vi "DisplayErrorsForDevice.vi"(0 "CmdLib In":refnum<k24>, 1 "Device Key":string, 2 "Device Address":i32, 3 "Prefix":string, 4 "Status:":refnum<vi>, 5 "error in":errorcluster) -> (14 "CmdLib Out":refnum<k24>, 15 "DeviceKey Out":string, 16 "Device Address Out":i32, 19 "error out":errorcluster)   [LabVIEW 2019]
uses:
  C:/Users/jyxks/OneDrive/Documents/Program Files/New Focus/New Focus Picomotor Application/Samples/LabVIEW/Model 8742/LabVIEW 2009/CmdLib.dll
  Program Files/New Focus/New Focus Picomotor Application/Samples/LabVIEW/Model 8742/LabVIEW 2009/CmdLib.dll
  <vilib>/regexp/Match Regular Expression.xnode
panel:
  in  "errMsg":string
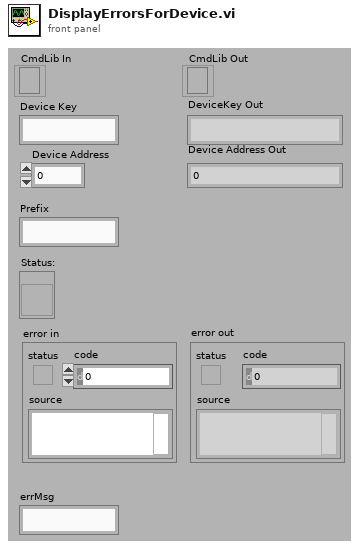
[diagram p1: front panel]
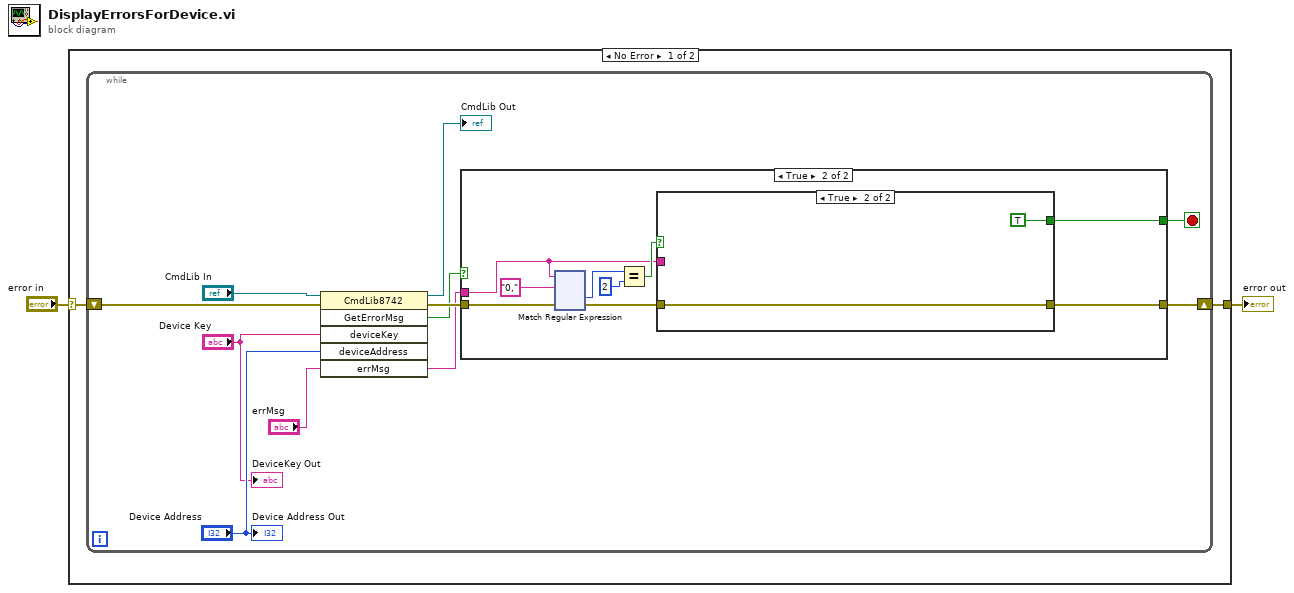
[diagram p0: block diagram]
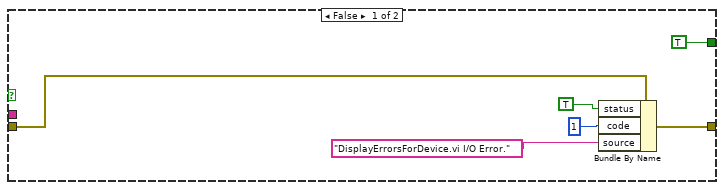
[diagram p2: hidden frame]
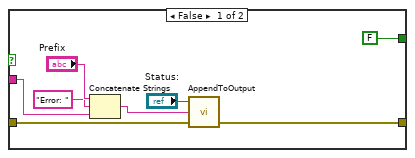
[diagram p3: hidden frame]
diagram:
  n1 = case shown="No Error" "error in" {
    selector: "error in" -> [w4 w155]
    tunnel: [w3 w155] -> w1
    frame No Error {
      n2 = while {
        shift-right: [w12] -> w3
        shift-left: w4 -> [w13]
        stop <- w5 stop-if-true
        n3 = invoke class="CmdLib8742" method="GetErrorMsg"(reference="CmdLib In", error in=w13, "deviceKey"="Device Key", "deviceAddress"="Device Address", "errMsg"="errMsg") -> (reference out=→"CmdLib Out":refnum<k24>, error out=w14:errorcluster, "GetErrorMsg"=w6:bool, "errMsg"=w7:string)  [unwired: 1 in, 2 out]
        n4 = case shown="True" w6 {
          tunnel: w14 -> [w21 w27]
          tunnel: [w16 w22] -> w12
          tunnel: w7 -> [_ w23]
          tunnel: [TRUE w25] -> w5
          frame False {
            n5 = Bundle By Name(cluster=w21, "status"=TRUE, "code"=1, "source"="DisplayErrorsForDevice.vi I/O Error.") -> (w16:errorcluster)
          }
          frame True {
            n6 = xnode "Match Regular Expression"("input string"=w23, "regular expression"="0,", "error in"=w27) -> ("offset past match"=w29:i32, "error out"=w24:errorcluster)  [unwired: 3 in, 3 out]
            n7 = Equal?(x=w29, y=2) -> (x = y?=w26:bool)
            n8 = case shown="True" w26 {
              tunnel: [FALSE TRUE] -> w25
              tunnel: w24 -> [w33 w39]
              tunnel: w23 -> [w32 _]
              tunnel: [w31 w39] -> w22
              frame False {
                n9 = Concatenate Strings("Prefix", "Error: ", w32) -> (w38:string)
                n10 = call "AppendToOutput.vi"("error in"=w33, "Input String"=w38, "Output Refnum In"="Status:") -> ("error out"=w31:errorcluster)  [unwired: 1 in, 1 out]
              }
              frame True {
              }
            }
          }
        }
        "DeviceKey Out" <- "Device Key"
        "Device Address Out" <- "Device Address"
      }
    }
    frame Error {
    }
  }
  "error out" <- w1
